vi "Test - Convert To 1D And Back.vi"() -> ()   [LabVIEW 2020, in "3D (FPGA).lvlib"]
uses:
  3D (FPGA).lvlib
panel:
  out "2D Pixel Data out":u32[][](array[numeric])
  in  "Array":u32[][](array[numeric])=[[1, 2, 3, 4, 5], [0, 0, 0, 0, 0], [0, 0, 0, 0, 0], [0, 0, 0, 0, 0], [0, 0, 0, 0, 0], [9, 10, 11, 12, 13]]
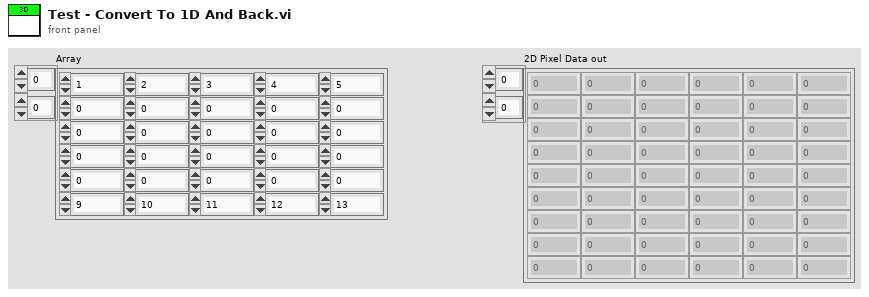
[diagram p1: front panel]
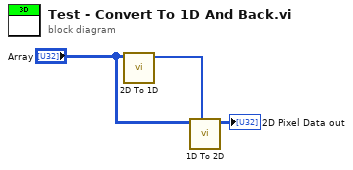
[diagram p0: block diagram]
diagram:
  n1 = call "2D To 1D.vi"("Pixel Data in"="Array") -> ("1D Pixel Data out"=w2:u32[])  [unwired: 10 in]
  n2 = call "1D To 2D.vi"("1D Pixel Data in"=w2, "2D Pixel Data in"="Array") -> ("2D Pixel Data out"=→"2D Pixel Data out":u32[][])  [unwired: 9 in]
